vi "Read key.vi"(8 "error in (no error)":errorcluster, 11 "Object in":refnum<class "Object.lvclass">) -> (0 "error out":errorcluster, 2 "key":string, 3 "Object out":refnum<class "Object.lvclass">)   [LabVIEW 2015, in "NI_AWS_S3.lvlib" / "Object.lvclass"]
uses:
  Object.lvclass
  Object.lvclass/Object.ctl
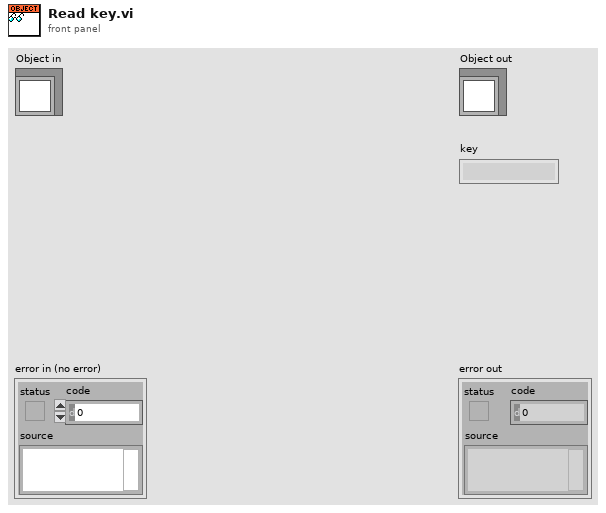
[diagram p1: front panel]
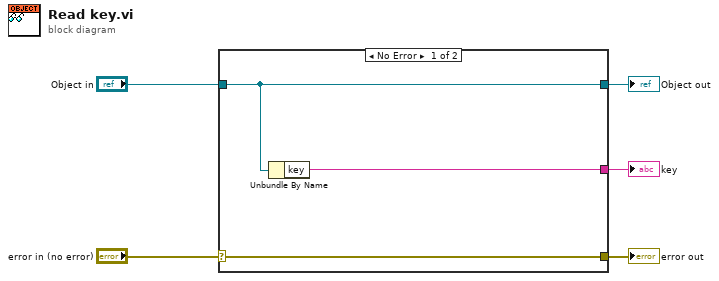
[diagram p0: block diagram]
diagram:
  n1 = case shown="No Error" "error in (no error)" {
    selector: "error in (no error)" -> [w8 w9]
    tunnel: [w8 w9] -> w4
    tunnel: [w7 w10] -> w2
    tunnel: "Object in" -> [w7 w10]
    tunnel: [w6 _] -> w1
    frame No Error {
      n2 = Unbundle By Name(w7) -> ("key"=w6:string)
    }
    frame Error {
    }
  }
  "error out" <- w4
  "Object out" <- w2
  "key" <- w1
